vi "Auto-Grab.vi"   [LabVIEW 2018]
uses:
  Implementation/Drive Operations.ctl
  Framework/Robot Global Data.vi
types:
  T1 = typedef "Command Status Info.ctl" = cluster{"Name":string, "Status":T2, "notifier out":T3}
  T2 = typedef "Completion Status.ctl" = enum16{"Successful", "Aborted", "Incomplete"}
  T3 = typedef "Completion Notifier.ctl" = refnum<notifier>
  T4 = cluster{"Reverse (T) / Normal (F)":bool, "Power Scaling (1=Normal) ":dbl, "Deadband Value":dbl}
  T5 = typedef "Drive Operations.ctl" = enum16{"Reserve", "Read Current", "Immediate", "J-Turn", "Play Back From Log", "Auto-Align"}
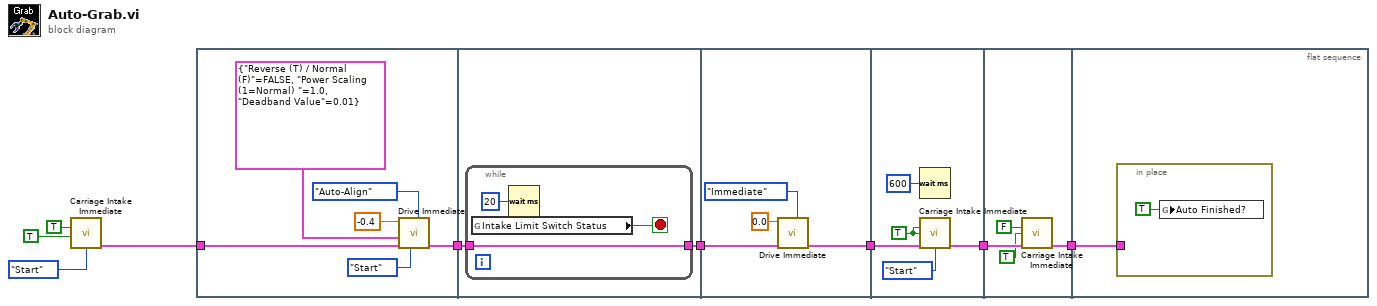
[diagram p0: block diagram]
diagram:
  n1 = call "Carriage Intake Immediate.vi"("Extend"=TRUE, "Close"=TRUE, "Synchronication"=enum16{"Start", "Wait"}."Start") -> ("Command Info Out"=w4:T1)  [unwired: 12 in]
  n2 = flat-sequence {
    tunnel: w4 -> [w12]
    tunnel: [w10] -> w9
    tunnel: w9 -> [w16]
    tunnel: [w17] -> w2
    tunnel: w2 -> [w24]
    tunnel: [w23] -> w1
    tunnel: w1 -> [w29]
    tunnel: [w28] -> w8
    tunnel: w8 -> [w33]
    tunnel: [w31] -> w7
    tunnel: w7 -> [w34]
    frame #0 {
      n3 = call "Drive Immediate.vi"("Operation"=Drive_Operations."Auto-Align", "Synchronication"=enum16{"Start", "Wait"}."Start", "Command Info In"=w12, "Modifiers"=T4 {"Reverse (T) / Normal (F)"=FALSE, "Power Scaling (1=Normal) "=1.0, "Deadband Value"=0.01}, "Left Setpoint (Power)"=-0.4) -> ("Command Info Out"=w10:T1)  [unwired: 6 in]
    }
    frame #1 {
      n4 = while {
        tunnel: [w20] -> w17
        tunnel: w16 -> [w20]
        stop <- w18 stop-if-true
        n5 = global read "Robot Global Data.vi" "Intake Limit Switch Status"() -> (w18:bool)
        n6 = Wait (ms)(milliseconds to wait=u32 20) -> ()  [unwired: 1 out]
      }
    }
    frame #2 {
      n7 = call "Drive Immediate.vi"("Operation"=Drive_Operations."Immediate", "Command Info In"=w24, "Left Setpoint (Power)"=0.0) -> ("Command Info Out"=w23:T1)  [unwired: 8 in]
    }
    frame #3 {
      w25 = TRUE ("Extend")
      n8 = Wait (ms)(milliseconds to wait=u32 600) -> ()  [unwired: 1 out]
      n9 = call "Carriage Intake Immediate.vi"("Extend"=w25, "Open"=w25, "Command Info In"=w29, "Synchronication"=enum16{"Start", "Wait"}."Start") -> ("Command Info Out"=w28:T1)  [unwired: 11 in]
    }
    frame #4 {
      n10 = call "Carriage Intake Immediate.vi"("Extend"=FALSE, "Open"=TRUE, "Command Info In"=w33) -> ("Command Info Out"=w31:T1)  [unwired: 12 in]
    }
    frame #5 {
      n11 = in-place {
        in-place-border: w34 -> [_]
        n12 = global write "Robot Global Data.vi" "Auto Finished?"(TRUE ("Auto Finished?")) -> ()
      }
    }
  }
